vi "save channels to stacked multi-tiff files.vi"(8 "frame number in":i32, 9 "last frame":bool, 11 "image data in":dbl[][](array[numeric])) -> ()   [LabVIEW 2012]
uses:
  Custom Controls/file format type def.ctl
  GFG/GFGpathGet.vi
  GFG/GFGnumericGet.vi
  Libtiff3/libtiff3.llb/libtiff3.lvlib
  GFG/GFG library.lvlib
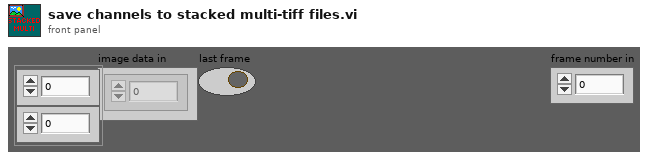
[diagram p1: front panel]
types:
  T1 = typedef "file format type def.ctl" = enum16{"16bit raw", "32bit raw", "16bit multi-tiff (interleave)", "16bit multi-tiff (separate)", "16bit multi-tiff (stacked)", "32bit multi-tiff (interleave)", "32bit multi-tiff (separate)", "32bit multi-tiff (stacked)", "16bit tiff series (interleave)", "16bit tiff series (separate)", "16bit tiff series (stacked)", "32bit tiff series (interleave)", "32bit tiff series (separate)", "32bit tiff series (stacked)"}
  T2 = cluster{"no..of.frames.to.acquire":dbl, "x.pixels":dbl, "y.pixels":dbl, "x.pixel.sz":dbl, "y.pixel.sz":dbl}
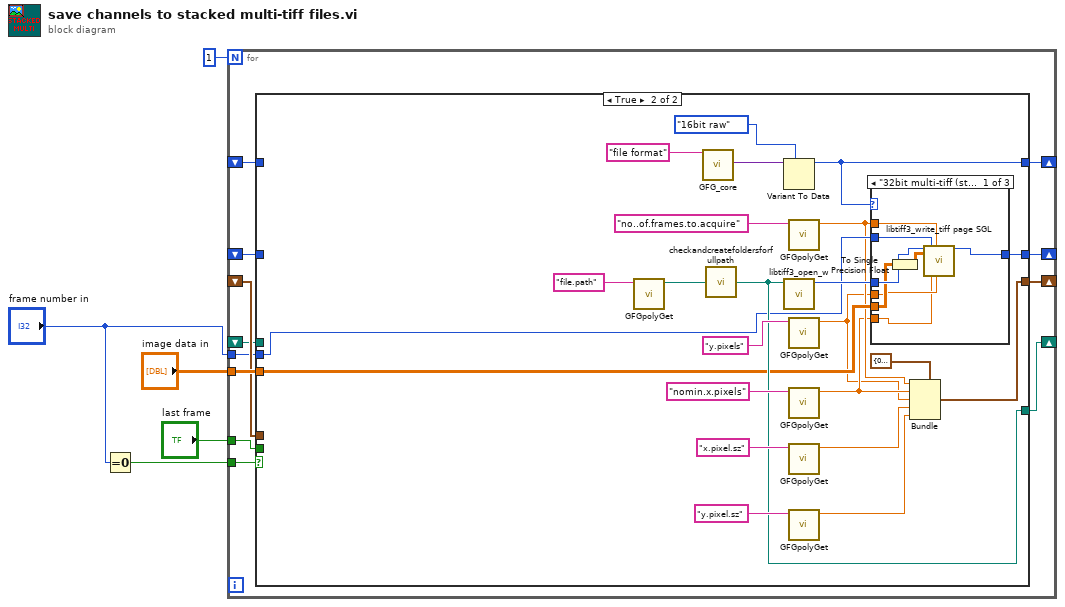
[diagram p0: block diagram]
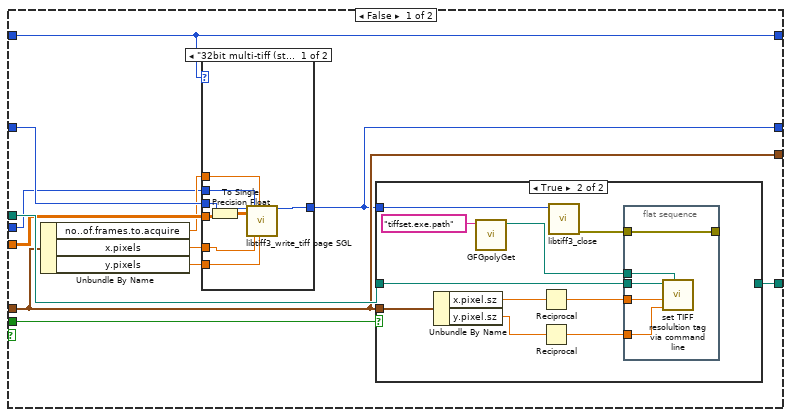
[diagram p2: hidden frame]
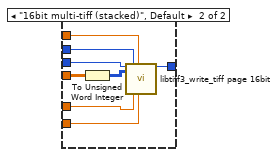
[diagram p3: hidden frame]
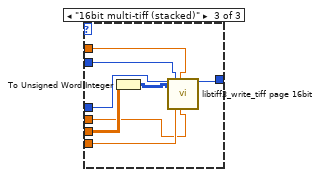
[diagram p6: hidden frame]
diagram:
  n1 = Equal To 0?(x="frame number in") -> (x = 0?=w4:bool)
  n2 = for {
    N: 1 -> [_]
    tunnel: w4 -> [w17]
    shift-right: [w16] -> _
    shift-left: _ -> [w15]
    tunnel: "image data in" -> [w14]
    shift-right: [w13] -> _
    shift-left: _ -> [w12]
    shift-right: [w11] -> _
    shift-left: _ -> [w10]
    shift-right: [w9] -> _
    shift-left: _ -> [w8]
    tunnel: "last frame" -> [w7]
    tunnel: "frame number in" -> [w6]
    n3 = case shown="True" w17 {
      tunnel: w12 -> [w20 _]
      tunnel: [w18 w64] -> w16
      tunnel: w15 -> [w26 _]
      tunnel: w14 -> [w27 w68]
      tunnel: [w20 w69] -> w13
      tunnel: [w19 w72] -> w11
      tunnel: w10 -> [w19 _]
      tunnel: [w25 w71] -> w9
      tunnel: w8 -> [w28 _]
      tunnel: w7 -> [w29 _]
      tunnel: w6 -> [w23 w66]
      frame False {
        n4 = Unbundle By Name(w19) -> ("no..of.frames.to.acquire"=w24:dbl, "x.pixels"=w22:dbl, "y.pixels"=w21:dbl)
        n5 = case shown="\"32bit multi-tiff (stacked)\"" w20 {
          tunnel: w27 -> [w33 w45]
          tunnel: w26 -> [w37 w43]
          tunnel: [w34 w42] -> w18
          tunnel: w24 -> [w35 w41]
          tunnel: w23 -> [w36 w40]
          tunnel: w22 -> [w32 w39]
          tunnel: w21 -> [w31 w38]
          frame "32bit multi-tiff (stacked)" {
            n6 = To Single Precision Float(number=w33) -> (single precision float=w30:sgl[][])
            n7 = call "libtiff3_write_tiff page SGL.vi"("Handle"=w37, "Image Pixels (Float)"=w30, "page"=w36, "x.pixels"=w32, "totalpages"=w35, "y.pixels"=w31) -> ("Handle out"=w34:i32)  [unwired: 12 in, 1 out]
          }
          frame "16bit multi-tiff (stacked)", Default {
            n8 = To Unsigned Word Integer(number=w45) -> (unsigned 16bit integer=w44:u16[][])
            n9 = call "libtiff3_write_tiff page 16bit.vi"("Handle"=w43, "Image Pixels (U16)"=w44, "page"=w40, "x.pixels"=w39, "totalpages"=w41, "y.pixels"=w38) -> ("Handle out"=w42:i32)  [unwired: 12 in, 1 out]
          }
        }
        n10 = case shown="True" w29 {
          tunnel: w19 -> [_ w51]
          tunnel: w28 -> [w46 w50]
          tunnel: w18 -> [_ w49]
          tunnel: [w46 _] -> w25
          frame False {
          }
          frame True {
            n11 = Unbundle By Name(w51) -> ("x.pixel.sz"=w52:dbl, "y.pixel.sz"=w53:dbl)
            n12 = call-poly "GFGpolyGet.vi"("Variable Name in"="tiffset.exe.path") -> ("Path"=w47:path)  [unwired: 9 in, 1 out]
            n13 = Reciprocal(x=w52) -> (1/x=w54:dbl)
            n14 = Reciprocal(x=w53) -> (1/x=w55:dbl)
            n15 = call "libtiff3_close.vi"("Handle"=w49) -> ("error out"=w56:errorcluster)  [unwired: 9 in]
            n16 = flat-sequence {
              tunnel: w50 -> [w61]
              tunnel: w56 -> [w58]
              tunnel: w54 -> [w60]
              tunnel: w55 -> [w59]
              tunnel: [w58] -> _
              tunnel: w47 -> [w57]
              frame #0 {
                n17 = call "set TIFF resolultion tag via command line.vi"("tiffset.exe file path"=w57, "y pixels per m"=w59, "x pixels per m"=w60, "TIFF file path"=w61) -> ()  [unwired: 8 in]
              }
            }
          }
        }
      }
      frame True {
        n18 = call-poly "GFGpolyGet.vi"("Variable Name in"="file.path") -> ("Path"=w70:path)  [unwired: 9 in, 1 out]
        n19 = call "GFG_core.vi"("Variable Name in"="file format") -> ("Variant Out"=w83:variant)  [unwired: 12 in, 6 out]
        n20 = call "checkandcreatefoldersforfullpath.vi"("Path IN"=w70) -> ("Path OUT"=w71:path)  [unwired: 4 in]
        n21 = Variant To Data(type=file_format_type_def."16bit raw" ("file format"), Variant=w83) -> (data=w69:T1)  [unwired: 1 in, 1 out]
        n22 = call "libtiff3_open_w.vi"("Input path"=w71) -> ("handle"=w67:i32)  [unwired: 9 in, 1 out]
        n23 = call-poly "GFGpolyGet.vi"("Variable Name in"="no..of.frames.to.acquire") -> ("Numeric"=w65:dbl)  [unwired: 9 in, 1 out]
        n24 = call-poly "GFGpolyGet.vi"("Variable Name in"="y.pixels" ("Tag in")) -> ("Numeric"=w62:dbl)  [unwired: 9 in, 1 out]
        n25 = call-poly "GFGpolyGet.vi"("Variable Name in"="nomin.x.pixels" ("Tag in")) -> ("Numeric"=w63:dbl)  [unwired: 9 in, 1 out]
        n26 = call-poly "GFGpolyGet.vi"("Variable Name in"="x.pixel.sz" ("Tag in")) -> ("Numeric"=w75:dbl)  [unwired: 9 in, 1 out]
        n27 = call-poly "GFGpolyGet.vi"("Variable Name in"="y.pixel.sz" ("Tag in")) -> ("Numeric"=w74:dbl)  [unwired: 9 in, 1 out]
        n28 = case shown="\"32bit multi-tiff (stacked)\"" w69 {
          tunnel: w68 -> [w88 _ w98]
          tunnel: w67 -> [w89 w93 w99]
          tunnel: w66 -> [w90 _ w100]
          tunnel: w65 -> [w91 _ w101]
          tunnel: [w92 w93 w94] -> w64
          tunnel: w63 -> [w85 _ w96]
          tunnel: w62 -> [w86 _ w95]
          frame "32bit multi-tiff (stacked)" {
            n29 = To Single Precision Float(number=w88) -> (single precision float=w87:sgl[][])
            n30 = call "libtiff3_write_tiff page SGL.vi"("Handle"=w89, "Image Pixels (Float)"=w87, "page"=w90, "x.pixels"=w85, "totalpages"=w91, "y.pixels"=w86) -> ("Handle out"=w92:i32)  [unwired: 12 in, 1 out]
          }
          frame Default {
          }
          frame "16bit multi-tiff (stacked)" {
            n31 = To Unsigned Word Integer(number=w98) -> (unsigned 16bit integer=w97:u16[][])
            n32 = call "libtiff3_write_tiff page 16bit.vi"("Handle"=w99, "Image Pixels (U16)"=w97, "page"=w100, "x.pixels"=w96, "totalpages"=w101, "y.pixels"=w95) -> ("Handle out"=w94:i32)  [unwired: 12 in, 1 out]
          }
        }
        n33 = Bundle(cluster=T2 {"no..of.frames.to.acquire"=0.0, "x.pixels"=0.0, "y.pixels"=0.0, "x.pixel.sz"=0.0, "y.pixel.sz"=0.0} ("output cluster"), "no..of.frames.to.acquire"=w65, "x.pixels"=w63, "y.pixels"=w62, "x.pixel.sz"=w75, "y.pixel.sz"=w74) -> (w72:T2)
      }
    }
  }
